vi "HapticSTM_flt.vi"() -> ()   [LabVIEW 2017]
uses:
  <vilib>/Analysis/3filter.llb/Filter Passband Type.ctl
  <vilib>/Utility/file.llb/Read Delimited Spreadsheet (DBL).vi
  SubVIs/GlobalClicksHeight_flt.vi
  <userlib>/HapticSTM/HapticSTM.lvlib
  <vilib>/ptbypt/NI_PtbyPt.lvlib
  <vilib>/Analysis/NI_AALBase.lvlib
panel:
  out "SeqString":string
  out "Seq":i32
  out "Raw and Scaled Z Positions":cluster{dbl, "Y":dbl}(graph)
  in  "Force Mode":u16(ring) items=["Exp Y", "Simple Log", "Linear", "Stacked Logs"]
  out "Button":bool
  out "Filtered Current":dbl
  in  "Reset Clicks":bool
  out "Scaled Force and Current":cluster{dbl, "Filtered x":dbl, dbl}(graph)
  in  "Maximum (pA)":dbl=9000.0
  in  "Setpoint (pA)":dbl=100.0
  out "PLANE HEIGHT":dbl
  out "Current":dbl
  out "Origin Y":dbl
  out "Origin X":dbl
  out "Output Z":dbl
  out "Nano Z":dbl
  out "Width":dbl
  out "VY":dbl
  out "VZ":dbl
  out "VX":dbl
  in  "STOP":bool
  in  "START":bool
  out "Fy":dbl
  out "Fz":dbl
  out "phi":dbl
  out "psi":dbl
  out "Fx":dbl
  out "theta":dbl
  out "x":dbl
  out "y":dbl
  out "z":dbl
  in  "Hardness":dbl=1.0
  out "Clicks":i32
  out "Height":dbl
  # "Frame"
  # "Position"
  # "Force"
  # "STM I/O"
  # "Angles"
  # "Current"
  # "Velocity"
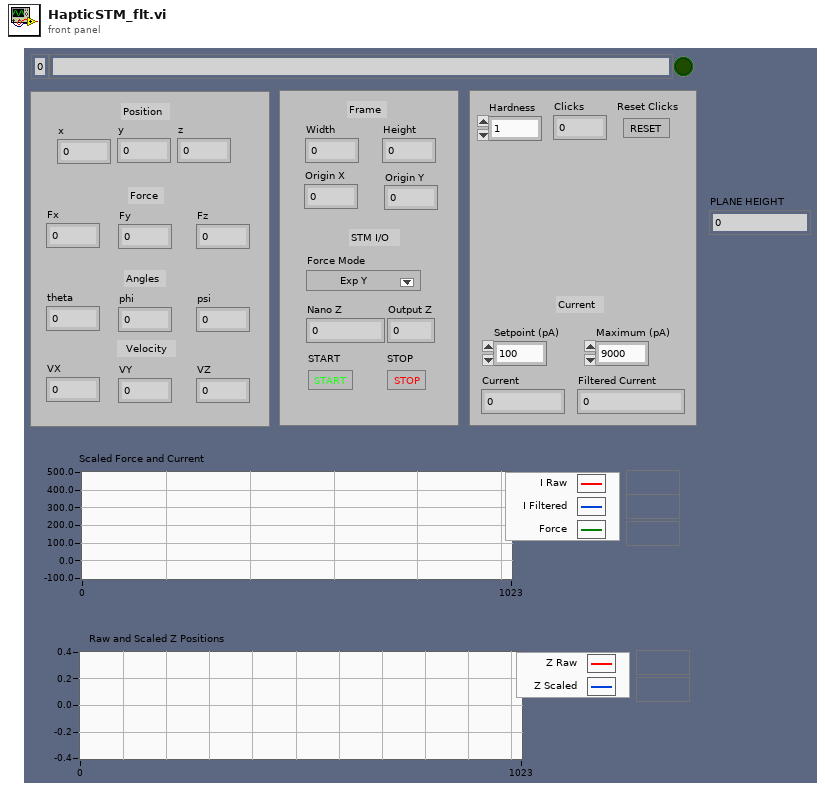
[diagram p1: front panel]
types:
  T1 = typedef "NI_AALBase.lvlib/Filter Passband Type.ctl" = enum32{"Lowpass", "Highpass", "Bandpass", "Bandstop"}
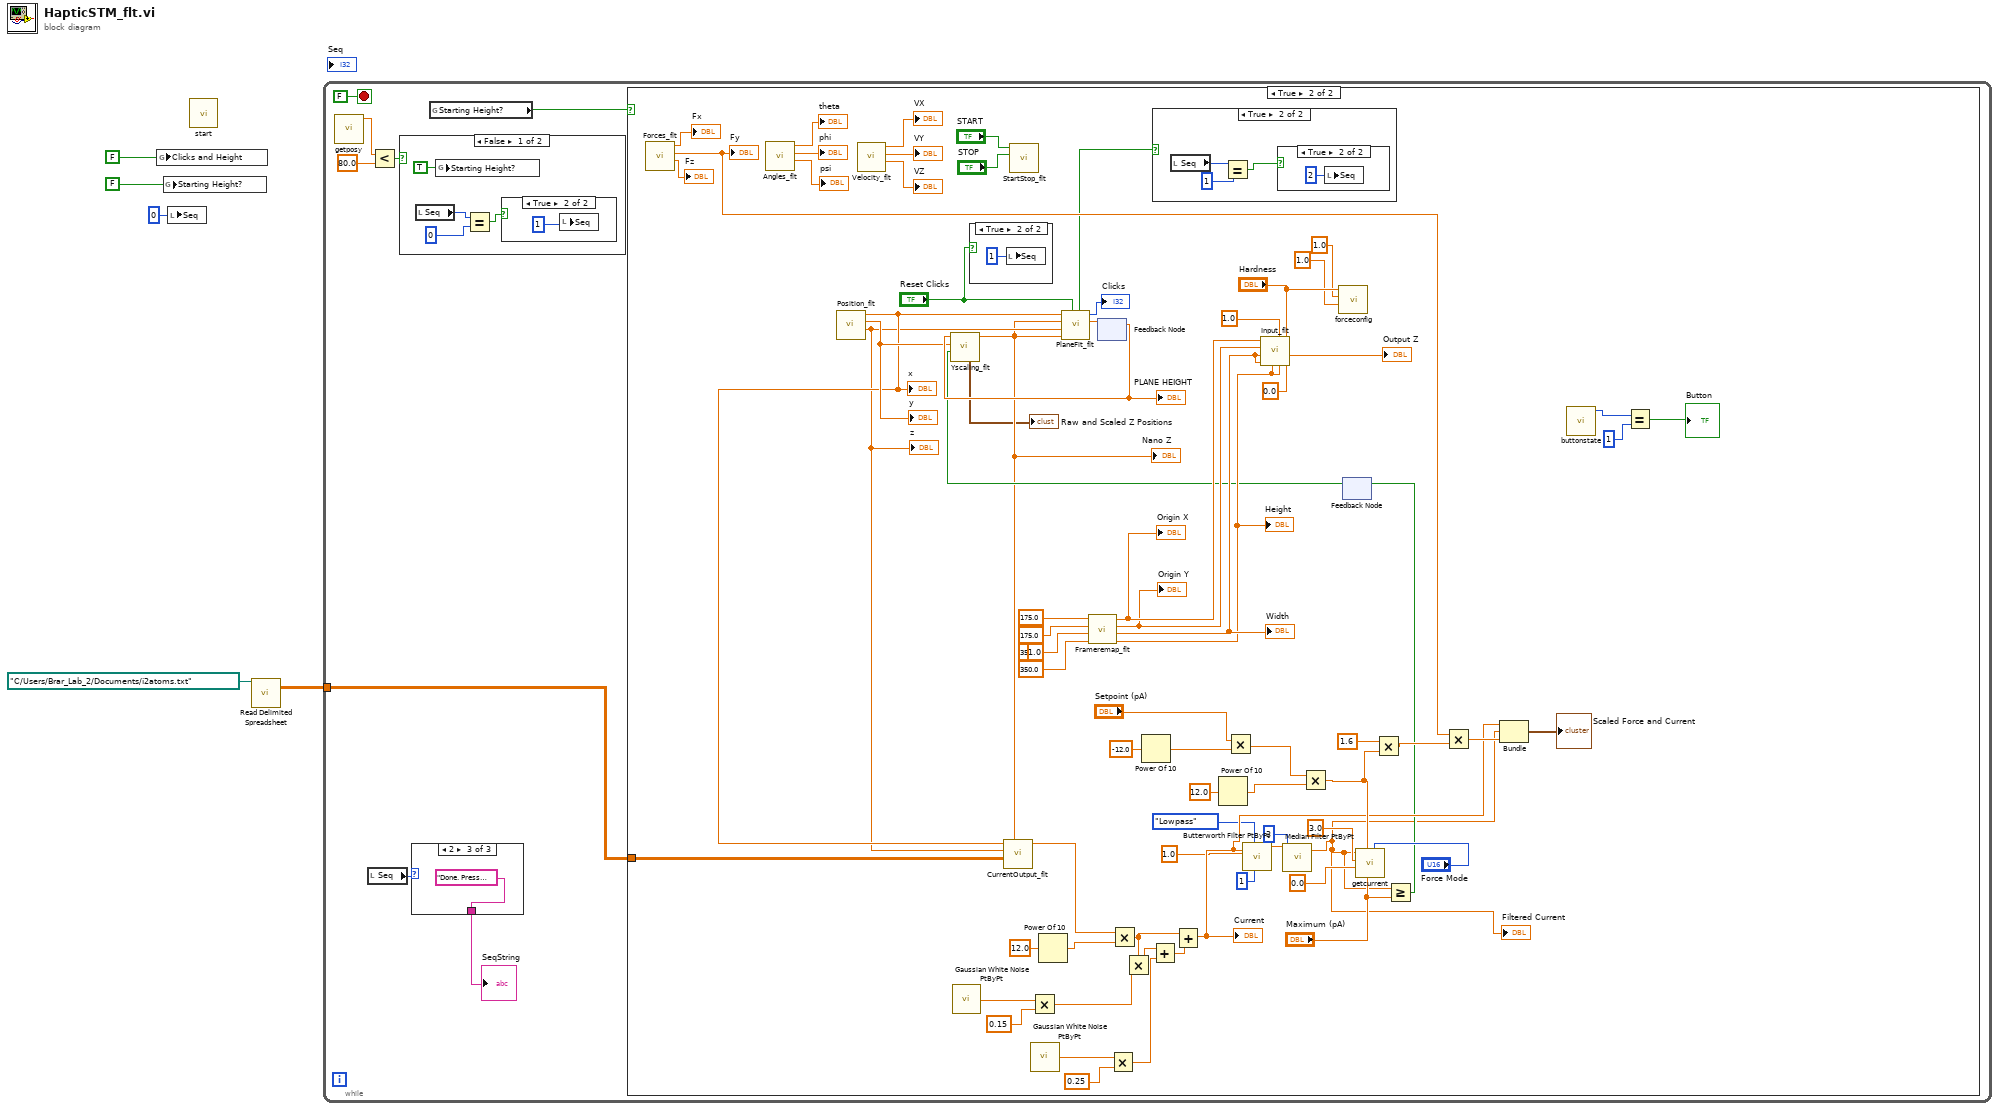
[diagram p0: block diagram]
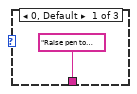
[diagram p2: hidden frame]
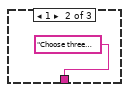
[diagram p3: hidden frame]
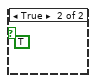
[diagram p5: hidden frame]
diagram:
  n1 = global write "GlobalClicksHeight_flt.vi" "Clicks and Height"(FALSE ("Clicks and Height")) -> ()
  n2 = global write "GlobalClicksHeight_flt.vi" "Starting Height?"(FALSE ("Clicks and Height")) -> ()
  n3 = local write "Seq"(0 ("Seq")) -> ()
  n4 = call <userlib>:"start.vi"() -> ()  [unwired: 11 in, 1 out]
  n5 = call-poly <vilib>:"Read Delimited Spreadsheet.vi"("file path (dialog if empty)"=path "C:/Users/Brar_Lab_2/Documents/i2atoms.txt") -> ("all rows"=w5:dbl[][])  [unwired: 9 in, 5 out]
  n6 = while {
    tunnel: w5 -> [w13]
    stop <- FALSE stop-if-true
    n7 = call <userlib>:"getposy.vi"() -> ("function return"=w12:dbl)  [unwired: 11 in]
    n8 = local read "Seq"() -> (w7:i32)
    n9 = Less?(x=w12, y=80.0) -> (x < y?=w10:bool)
    n10 = case shown="False" w10 {
      frame False {
        n11 = local read "Seq"() -> (w19:i32)
        n12 = global write "GlobalClicksHeight_flt.vi" "Starting Height?"(TRUE ("Starting Height?")) -> ()
        n13 = Equal?(x=w19, y=0) -> (x = y?=w17:bool)
        n14 = case shown="True" w17 {
          frame False {
          }
          frame True {
            n15 = local write "Seq"(1 ("Seq")) -> ()
          }
        }
      }
      frame True {
        (unwired) TRUE ("Clicks and Height")
      }
    }
    n16 = case shown="2" w7 {
      tunnel: ["Raise pen to begin." "Choose three points, then raise the arm to plane." "Done. Press 'STOP' to stop at anytime."] -> w6
      frame 0, Default {
      }
      frame 1 {
      }
      frame 2 {
      }
    }
    "SeqString" <- w6
    n17 = global read "GlobalClicksHeight_flt.vi" "Starting Height?"() -> (w9:bool)
    n18 = case shown="True" w9 {
      tunnel: w13 -> [_ w33]
      frame False {
      }
      frame True {
        (unwired) 1.0 ("FO X")
        n19 = call "Forces_flt.vi"() -> ("Fz"=→"Fz":dbl, "Fy"=w61:dbl, "Fx"=→"Fx":dbl)  [unwired: 9 in]
        "Fy" <- w61
        n20 = call "Angles_flt.vi"() -> ("psi"=→"psi":dbl, "phi"=→"phi":dbl, "theta"=→"theta":dbl)  [unwired: 9 in]
        n21 = call "Position_flt.vi"() -> ("Z"=w34:dbl, "Y"=w47:dbl, "X"=w35:dbl)  [unwired: 9 in]
        "x" <- w35
        "y" <- w47
        "z" <- w34
        n22 = call "Velocity_flt.vi"() -> ("VZ"=→"VZ":dbl, "VY"=→"VY":dbl, "VX"=→"VX":dbl)  [unwired: 9 in]
        n23 = call <vilib>:"Gaussian White Noise PtByPt.vi"() -> ("Gaussian white noise"=w60:dbl)  [unwired: 3 in]
        n24 = case shown="True" "Reset Clicks" {
          frame False {
          }
          frame True {
            n25 = local write "Seq"(1 ("Seq")) -> ()
          }
        }
        n26 = call "StartStop_flt.vi"("STOP"="STOP", "START"="START") -> ()  [unwired: 10 in]
        n27 = Multiply(x=w60, y=0.15) -> (x*y=w58:dbl)
        n28 = call <vilib>:"Gaussian White Noise PtByPt.vi"() -> ("Gaussian white noise"=w55:dbl)  [unwired: 3 in]
        n29 = Power Of 10(x=12.0) -> (10^x=w79:dbl)
        n30 = call "Frameremap_flt.vi"("FH"=350.0 ("FO X"), "FW"=350.0 ("FO X"), "FO Z"=175.0 ("FO X"), "FO X"=175.0) -> ("FH"=w84:dbl, "FW"=w85:dbl, "Z Origin"=w71:dbl, "X Origin"=w72:dbl)  [unwired: 4 in]
        "Height" <- w84
        "Width" <- w85
        "Origin X" <- w72
        "Origin Y" <- w71
        n31 = feedback #1() -> (w73:dbl)  [unwired: 1 in]
        "PLANE HEIGHT" <- w73
        n32 = Multiply(x=w55, y=0.25) -> (x*y=w51:dbl)
        n33 = Power Of 10(x=-12.0) -> (10^x=w68:dbl)
        n34 = Power Of 10(x=12.0) -> (10^x=w70:dbl)
        n35 = Multiply(x="Setpoint (pA)", y=w68) -> (x*y=w66:dbl)
        n36 = call "Input_flt.vi"("Current * 10^input"=0.0, "Sensitivity"="Hardness", "Scopez"=w84, "Drag"=1.0, "FH"=w84, "FW"=w85, "Scopex"=w85, "Z origin"=w71, "X origin"=w72) -> ("Scaled Current"=→"Output Z":dbl)  [unwired: 2 in]
        n37 = Multiply(x=w66, y=w70) -> (x*y=w48:dbl)
        n38 = call <userlib>:"forceconfig.vi"("c"=1.0, "b"=1.0, "a"="Hardness") -> ()  [unwired: 9 in]
        n39 = feedback #2() -> (w64:bool)  [unwired: 1 in]
        n40 = call "Yscaling_flt.vi"("Current Maxed?"=w64, "Y"=w47, "Plane Height"=w73) -> ("y scaled"=w32:dbl, "Zpos Graph (nm)"=→"Raw and Scaled Z Positions":cluster{dbl, "function return":dbl})  [unwired: 7 in]
        "Nano Z" <- w32
        n41 = call "CurrentOutput_flt.vi"("y scaled"=w32, "array"=w33, "Z Input"=w34, "X Input"=w35) -> ("Current Out"=w36:dbl)  [unwired: 7 in]
        n42 = call "PlaneFit_flt.vi"("Reset Clicks"="Reset Clicks", "Y PEN"=w32, "Z"=w34, "Nano Z"=w32, "X"=w35) -> ("Plane Height (m)"=w82:dbl, "Clicks"=→"Clicks":i32, "Planing Done?"=w27:bool)  [unwired: 4 in]
        n43 = feedback-in #1(w82) -> ()
        n44 = Multiply(x=w36, y=w79) -> (x*y=w57:dbl)
        n45 = Multiply(x=w57, y=w58) -> (x*y=w52:dbl)
        n46 = Add(x=w52, y=w51) -> (x+y=w53:dbl)
        n47 = case shown="True" w27 {
          frame False {
          }
          frame True {
            n48 = local read "Seq"() -> (w100:i32)
            n49 = Equal?(x=w100, y=1) -> (x = y?=w98:bool)
            n50 = case shown="True" w98 {
              frame False {
              }
              frame True {
                n51 = local write "Seq"(2 ("Seq")) -> ()
              }
            }
          }
        }
        n52 = Add(x=w57, y=w53) -> (x+y=w43:dbl)
        "Current" <- w43
        n53 = call <vilib>:"Butterworth Filter PtByPt.vi"("order"=1, "filter type"=Filter_Passband_Type."Lowpass", "sampling freq: fs"=1.0, "x"=w43) -> ("Filtered x"=w39:dbl)  [unwired: 5 in, 1 out]
        n54 = call <vilib>:"Median Filter PtByPt.vi"("rank"=3, "x"=w39) -> ("Filtered x"=w24:dbl)  [unwired: 2 in, 1 out]
        "Filtered Current" <- w24
        n55 = call <userlib>:"getcurrent.vi"("forcemode"="Force Mode", "maxcurrentin"="Maximum (pA)", "setpoint"=w48, "minforcey"=0.0, "maxforcey"=3.0, "currentin"=w24) -> ()  [unwired: 6 in]
        n56 = Multiply(x=1.6 ("y"), y=w48) -> (x*y=w49:dbl)
        n57 = Greater Or Equal?(x=w24, y="Maximum (pA)") -> (x >= y?=w31:bool)
        n58 = feedback-in #2(w31) -> ()
        n59 = Multiply(x=w61, y=w49) -> (x*y=w56:dbl)
        n60 = Bundle(w43, "Filtered x"=w24, w56) -> (→"Scaled Force and Current":cluster{dbl, "Filtered x":dbl, dbl})  [unwired: 1 in]
        n61 = call <userlib>:"buttonstate.vi"() -> ("function return"=w46:i32)  [unwired: 11 in]
        n62 = Equal?(x=w46, y=1) -> (x = y?=→"Button":bool)
      }
    }
  }
